vi "StopAcquisition.vi"(8 "error in (no error)":errorcluster, 11 "Camera_Prime95B in":refnum<class "Camera_Prime95B.lvclass">) -> (0 "error out":errorcluster, 3 "Camera_Prime95B out":refnum<class "Camera_Prime95B.lvclass">)   [LabVIEW 2020, in "Camera_Prime95B.lvlib" / "Camera_Prime95B.lvclass"]
uses:
  Camera_Prime95B.lvclass
  Hardware Abstraction Layer/Component/Device/Device/DeviceStatus.ctl
  Camera_Prime95B.lvclass/Camera_Prime95B.ctl
  E:/Development/DevHardSoftware/MicroscopyFramework/Model/Hardware Layer/Real Hardware/Camera_Prime95B/Camera_Prime95B/Dependencies/PVCamNET.dll
  Dependencies/PVCamNET.dll
  Hardware Abstraction Layer/Component/Camera/Camera/Camera.lvclass
  Hardware Abstraction Layer/Component/Device/Device/Device.lvlib
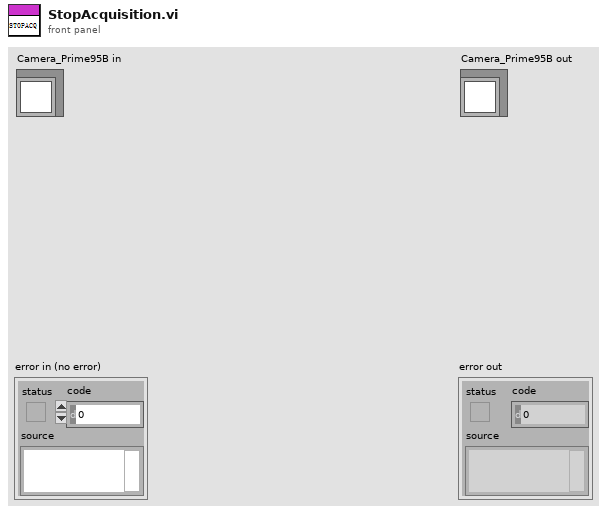
[diagram p1: front panel]
types:
  T1 = typedef "Device.lvlib/DeviceStatus.ctl" = i32
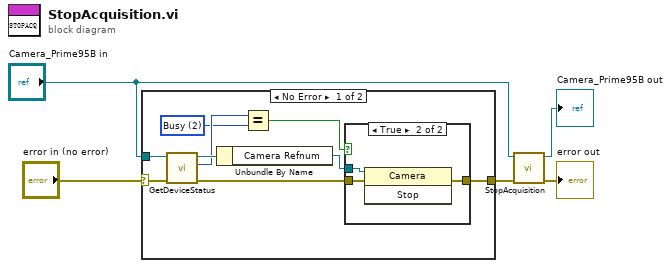
[diagram p0: block diagram]
diagram:
  n1 = case shown="No Error" "error in (no error)" {
    selector: "error in (no error)" -> [w12 w19]
    tunnel: [w14 w19] -> w2
    tunnel: "Camera_Prime95B in" -> [w10 _]
    frame No Error {
      w6 = T1 2 items=["Offline", "Idle", "Busy"] ("y")
      n2 = call-dynamic "GetDeviceStatus.vi"("error in (no error)"=w12, "Camera_Prime95B in"=w10) -> ("error out"=w11:errorcluster, "Status"=w8:T1, "Camera_Prime95B out"=w9:refnum<class "Camera_Prime95B.lvclass">)  [unwired: 7 in]
      n3 = Unbundle By Name(w9) -> ("Camera Refnum"=w13:refnum<k24>)
      n4 = Equal?(x=w8, y=w6) -> (x = y?=w7:bool)
      n5 = case shown="True" w7 {
        tunnel: [w15 w18] -> w14
        tunnel: w11 -> [w15 w17]
        tunnel: w13 -> [_ w16]
        frame False {
        }
        frame True {
          n6 = invoke class="Camera" method="Stop"(reference=w16, error in=w17) -> (error out=w18:errorcluster)  [unwired: 1 in, 2 out]
        }
      }
    }
    frame Error {
    }
  }
  n7 = call-parent "StopAcquisition.vi"("error in (no error)"=w2, "Device in"="Camera_Prime95B in") -> ("error out"=→"error out":errorcluster, "Device out"=→"Camera_Prime95B out":refnum<class "Camera_Prime95B.lvclass">)  [unwired: 8 in]
